vi "WLAN_FrameAnalysis_BothMessages - 3 SC.vi"(8 "error in (no error)":errorcluster, 11 "input cluster":cluster{"t0":dbl, "dt":dbl, "Y":cdb[]}) -> (0 "error out":errorcluster, 1 "Constellation":cdb[](graph), 2 "Modulation parameter":T1, 3 "SC Bits":i8[](array[numeric]), 4 "Frequency offset":dbl, 5 "SIG valid?":bool, 6 "SC Bits 2":i8[](array[numeric]), 7 "Base Bits":i8[](array[numeric]))   [LabVIEW 2022 SP3]
panel:
  out "Constellation 3":cdb[](graph)
  out "Constellation 2":cdb[](graph)
  out "x+y":dbl
  out "Frequency offset(LTF)":dbl
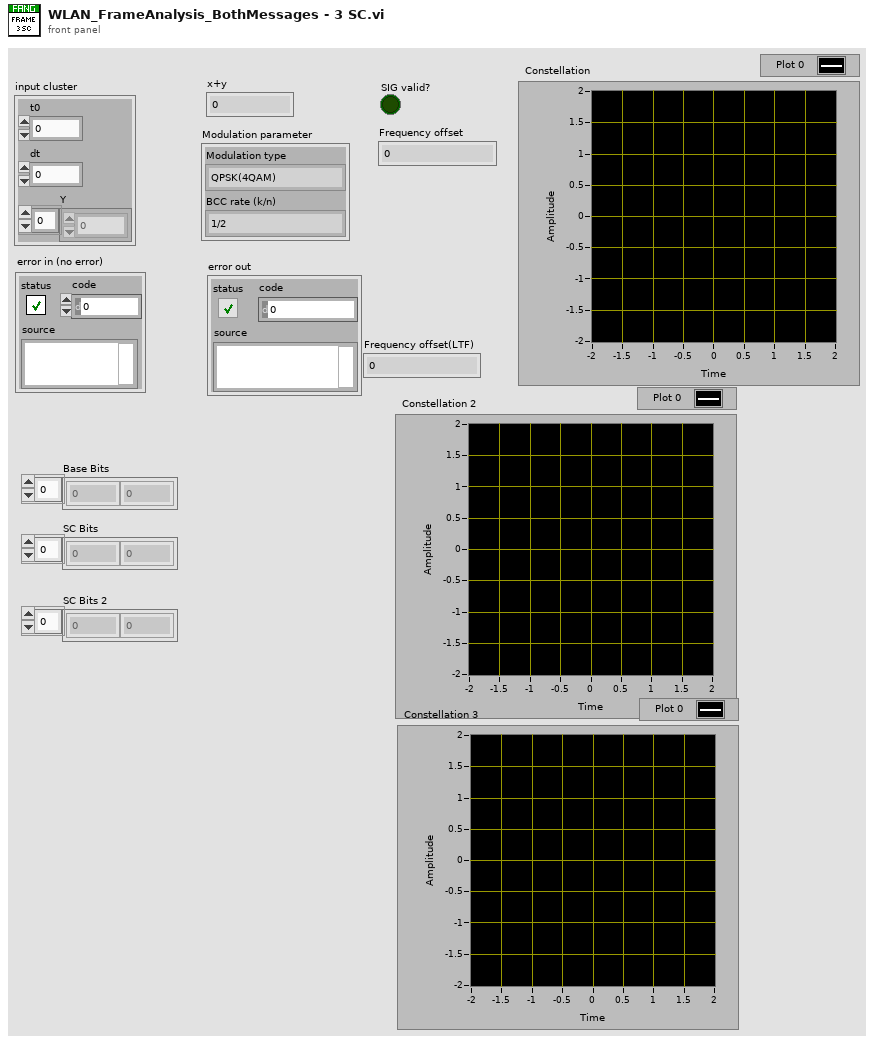
[diagram p1: front panel]
types:
  T1 = cluster{"Modulation type":enum16{"QPSK(4QAM)", "64QAM", "16QAM", "BPSK"}, "BCC rate (k/n)":enum16{"1/2", "2/3", "3/4"}}
  T2 = enum16{"QPSK(4QAM)", "64QAM", "16QAM", "BPSK", "BPSK Vertical"}
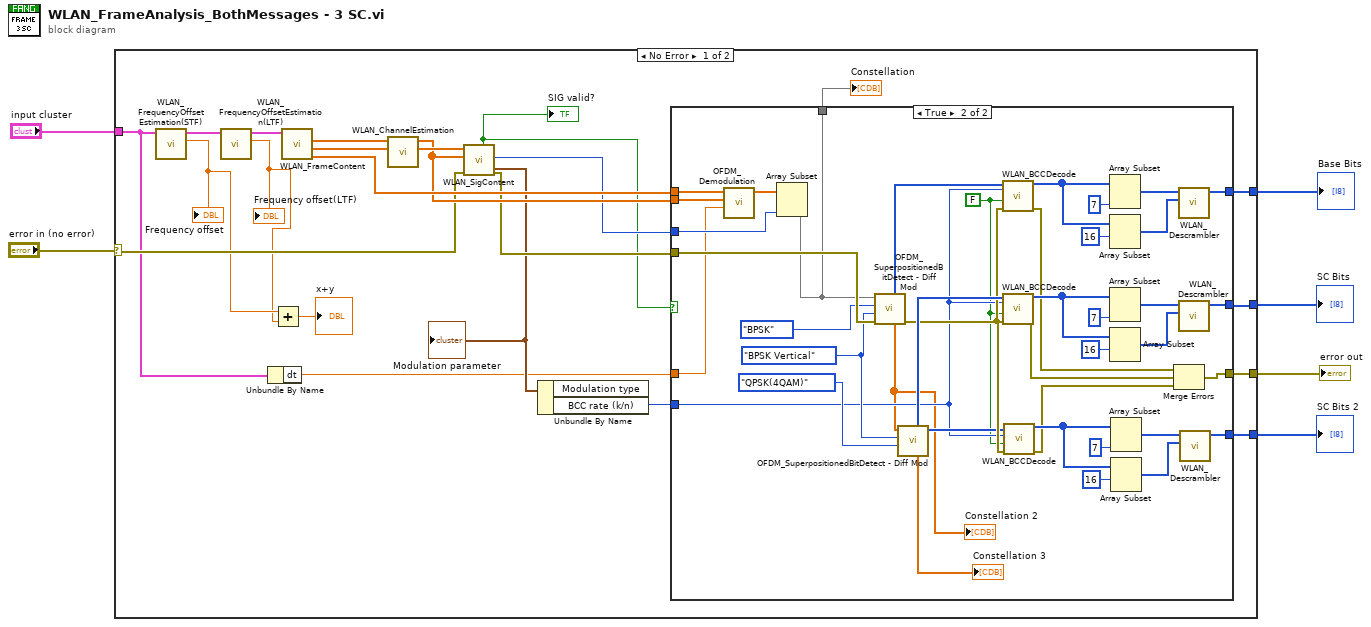
[diagram p0: block diagram]
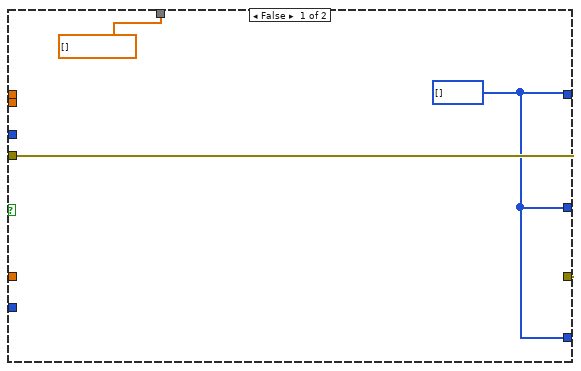
[diagram p2: hidden frame]
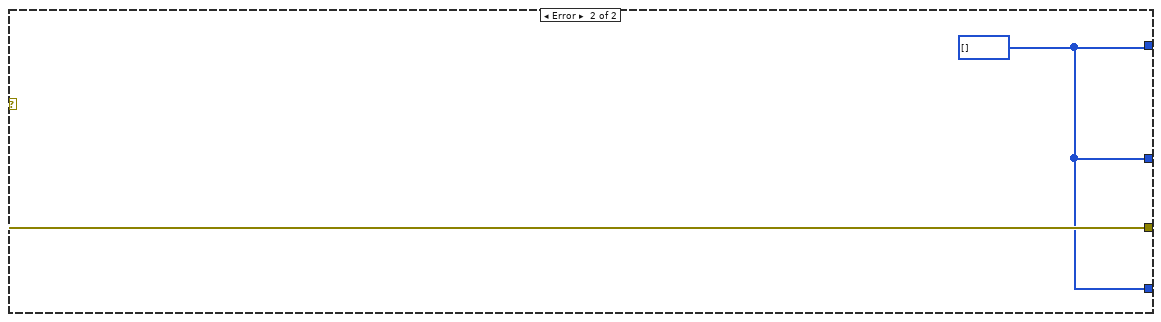
[diagram p3: hidden frame]
diagram:
  n1 = case shown="No Error" "error in (no error)" {
    selector: "error in (no error)" -> [w16 w73]
    tunnel: "input cluster" -> [w10 _]
    tunnel: [w22 w73] -> w5
    tunnel: [w21 w72] -> w4
    tunnel: [w8 w72] -> w2
    tunnel: [w7 w72] -> w1
    frame No Error {
      n2 = call "WLAN_FrequencyOffsetEstimation(STF).vi"("output cluster"=w10) -> ("Frequency offset(STF)"=w14:dbl, "output cluster 2"=w15:cluster{"t0":dbl, "dt":dbl, "Y":cdb[]})  [unwired: 8 in]
      "Frequency offset" <- w14
      n3 = call "WLAN_FrequencyOffsetEstimation(LTF).vi"("input cluster"=w15) -> ("Frequency offset(LTF)"=w13:dbl, "output cluster"=w11:cluster{"t0":dbl, "dt":dbl, "Y":cdb[]})  [unwired: 9 in]
      "Frequency offset(LTF)" <- w13
      n4 = Unbundle By Name(w10) -> ("dt"=w9:dbl)
      n5 = Add(x=w14, y=w13) -> (x+y=→"x+y":dbl)
      n6 = call "WLAN_FrameContent.vi"("Input cluster"=w11) -> ("DATA"=w28:cdb[], "SIG"=w26:cdb[], "LTF"=w27:cdb[])  [unwired: 7 in, 1 out]
      n7 = call "WLAN_ChannelEstimation.vi"("LTF"=w27) -> ("Frequency estimation"=w25:cdb[])  [unwired: 10 in]
      n8 = call "WLAN_SigContent.vi"("error in (no error)"=w16, "Frequency channel estimation"=w25, "SIG"=w26) -> ("error out"=w24:errorcluster, "Symbol numbers"=w23:i32, "Modulation parameter"=w20:T1, "SIG valid?"=w17:bool)  [unwired: 3 in, 2 out]
      "Modulation parameter" <- w20
      "SIG valid?" <- w17
      n9 = Unbundle By Name(w20) -> ("BCC rate (k/n)"=w19:enum16{"1/2", "2/3", "3/4"})  [unwired: 1 out]
      n10 = case shown="True" w17 {
        tunnel: w28 -> [_ w71]
        tunnel: [w31 w43] -> w22
        tunnel: w25 -> [_ w69]
        tunnel: w24 -> [w31 w68]
        tunnel: w23 -> [_ w67]
        tunnel: [w29 w60] -> w21
        tunnel: w19 -> [_ w36]
        tunnel: [cdb[] [] w62] -> w18
        tunnel: w9 -> [_ w59]
        tunnel: [w29 w52] -> w8
        tunnel: [w29 w34] -> w7
        frame False {
          w29 = i8[] [] ("scrambled bits")
        }
        frame True {
          w39 = T2."BPSK Vertical" ("Modulation type")
          w35 = FALSE ("need add zeros?")
          n11 = call "OFDM_Demodulation.vi"("sampling period"=w59, "Frequency channel estimation"=w69, "Input sequence"=w71) -> ("Output sequence"=w70:cdb[])  [unwired: 7 in, 1 out]
          n12 = Array Subset(array=w70, length=w67) -> (w62:cdb[])  [unwired: 1 in]
          n13 = call "OFDM_SuperpositionedBitDetect - Diff Mod.vi"("Input symbols"=w62, "Modulation type"=T2."BPSK", "Modulation type 2"=w39, "error in (no error)"=w68) -> ("Base Bits"=w53:i8[], "SC Symbols"=w33:cdb[], "error out"=w41:errorcluster)  [unwired: 3 in, 1 out]
          "Constellation 2" <- w33
          n14 = call "OFDM_SuperpositionedBitDetect - Diff Mod.vi"("Input symbols"=w33, "Modulation type"=w39, "Modulation type 2"=T2."QPSK(4QAM)" ("Modulation type")) -> ("Base Bits"=w49:i8[], "SC Symbols"=→"Constellation 3":cdb[], "SC Bits"=w37:i8[])  [unwired: 4 in, 1 out]
          n15 = call "WLAN_BCCDecode.vi"("error in (no error)"=w41, "need add zeros?"=w35, "BCC rate (k/n)"=w36, "input bit stream"=w53) -> ("error out"=w50:errorcluster, "output bit stream"=w58:i8[])  [unwired: 6 in]
          n16 = call "WLAN_BCCDecode.vi"("error in (no error)"=w41, "need add zeros?"=w35, "BCC rate (k/n)"=w36, "input bit stream"=w49) -> ("error out"=w51:errorcluster, "output bit stream"=w61:i8[])  [unwired: 6 in]
          n17 = call "WLAN_BCCDecode.vi"("error in (no error)"=w41, "need add zeros?"=w35, "BCC rate (k/n)"=w36, "input bit stream"=w37) -> ("error out"=w42:errorcluster, "output bit stream"=w44:i8[])  [unwired: 6 in]
          n18 = Array Subset(array=w58, length=7) -> (w57:i8[])  [unwired: 1 in]
          n19 = Array Subset(array=w58, index=16) -> (w56:i8[])  [unwired: 1 in]
          n20 = Array Subset(array=w61, length=7) -> (w63:i8[])  [unwired: 1 in]
          n21 = Array Subset(array=w61, index=16) -> (w64:i8[])  [unwired: 1 in]
          n22 = Array Subset(array=w44, length=7) -> (w45:i8[])  [unwired: 1 in]
          n23 = Array Subset(array=w44, index=16) -> (w46:i8[])  [unwired: 1 in]
          n24 = Merge Errors(w50, w51, w42) -> (w43:errorcluster)
          n25 = call "WLAN_Descrambler.vi"("scrambler initial bits"=w57, "data bits"=w56) -> ("scrambled bits"=w52:i8[])  [unwired: 7 in]
          n26 = call "WLAN_Descrambler.vi"("scrambler initial bits"=w63, "data bits"=w64) -> ("scrambled bits"=w60:i8[])  [unwired: 7 in]
          n27 = call "WLAN_Descrambler.vi"("scrambler initial bits"=w45, "data bits"=w46) -> ("scrambled bits"=w34:i8[])  [unwired: 7 in]
        }
      }
      "Constellation" <- w18
    }
    frame Error {
      w72 = i8[] [] ("scrambled bits")
    }
  }
  "error out" <- w5
  "SC Bits" <- w4
  "Base Bits" <- w2
  "SC Bits 2" <- w1
